vi "Scale Value FGV.vi"(7 "Write":bool, 8 "error in (no error)":errorcluster, 11 "Scale In (g)":dbl) -> (0 "error out":errorcluster, 3 "Scale Out (g)":dbl)   [LabVIEW 2018]
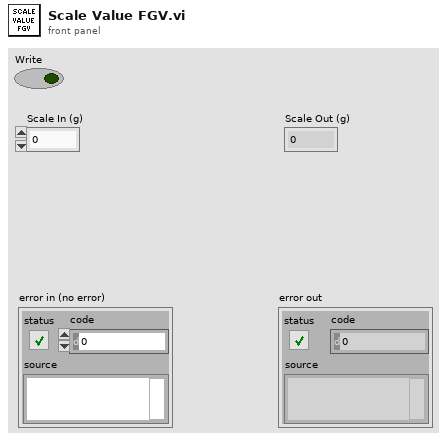
[diagram p1: front panel]
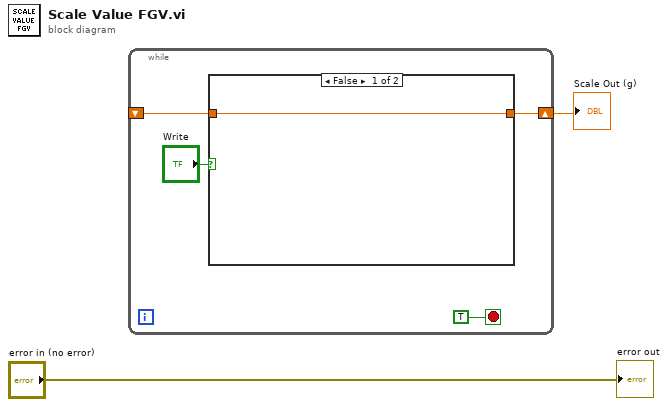
[diagram p0: block diagram]
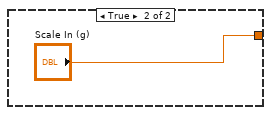
[diagram p2: hidden frame]
diagram:
  n1 = while {
    shift-right: [w4] -> w2
    shift-left: _ -> [w3]
    stop <- TRUE stop-if-true
    n2 = case shown="False" "Write" {
      tunnel: [w7 "Scale In (g)"] -> w4
      tunnel: w3 -> [w7 _]
      frame False {
      }
      frame True {
      }
    }
  }
  "Scale Out (g)" <- w2
  "error out" <- "error in (no error)"
